vi "Update Plot Name.vi"(8 "error in (no error)":errorcluster, 10 "NewVal":cluster{"String":string, "Picture":picture}[](array[cluster]), 11 "2D Error Bar.lvclass in":refnum<class "2D Error Bar.lvclass">) -> (0 "error out":errorcluster, 3 "2D Error Bar.lvclass out":refnum<class "2D Error Bar.lvclass">)   [LabVIEW 2017, in "2D Error Bar.lvclass"]
uses:
  <vilib>/Math Plots/2D Math Plots/2D Error Bar/2D Error Bar/2D Error Bar.lvclass
  <vilib>/Math Plots/2D Math Plots/2D Error Bar/2D Error Bar/2D Error Bar.lvclass/2D Error Bar.ctl
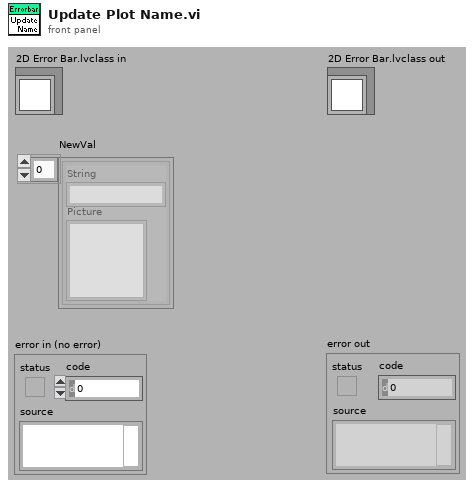
[diagram p1: front panel]
types:
  T1 = typedef "2D Plot.lvclass/Plot Property Array.ctl" = T2[]
  T2 = typedef "2D Plot.lvclass/Plot Property.ctl" = cluster{"Bar Plot Style":u8, "DigitalLineStyle":u8, "TransitionLocation":u8, "Transition Type":u8, "Fill To":i16, "Fill/Pt. Color":u32, "Label Style":u8, "Line Style":u8, "Line Width":u8, "Plot Color":u32, "Plot Interpolation":u8, "Plot Name":string, "Point Style":u8, "Visible?":bool, "XScaleIdx":u32, "YScaleIdx":u32}
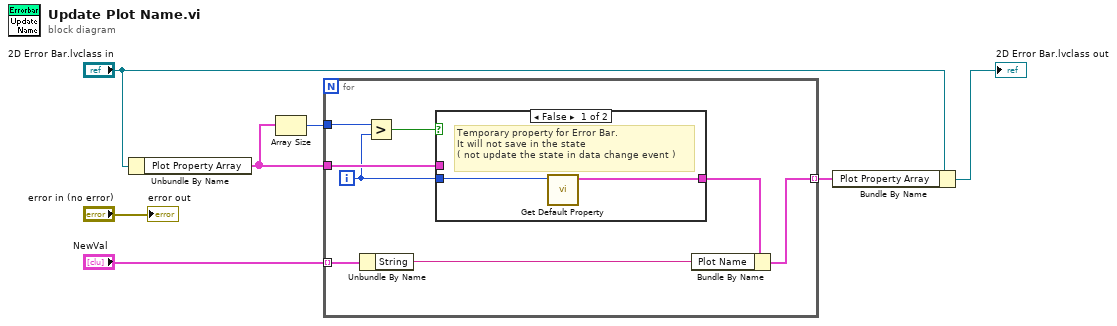
[diagram p0: block diagram]
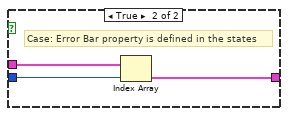
[diagram p2: hidden frame]
diagram:
  n1 = Unbundle By Name("2D Error Bar.lvclass in") -> ("Plot Property Array"=w6:T1)
  n2 = Array Size(array=w6) -> (size(s)=w7:i32)
  n3 = for {
    tunnel: "NewVal" -> [w14] mode=indexing
    tunnel: w6 -> [w10]
    tunnel: [w15] -> w5 mode=indexing
    tunnel: w7 -> [w11]
    i -> [w8]
    n4 = Unbundle By Name(w14) -> ("String"=w13:string)
    n5 = Greater?(x=w11, y=w8) -> (0:w12:bool)
    n6 = case shown="False" w12 {
      tunnel: w10 -> [_ w20]
      tunnel: w8 -> [w17 w19]
      tunnel: [w16 w18] -> w9
      frame False {
        # "Temporary property for Error Bar.\nIt will not save in the state\n( not update the state in data change event )"
        n7 = call <vilib>:"Get Default Property.vi"("Index"=w17) -> ("Temporary Property"=w16:T2)  [unwired: 3 in, 7 out]
      }
      frame True {
        # "Case: Error Bar property is defined in the states"
        n8 = Index Array(array=w20, index=w19) -> (element=w18:T2)
      }
    }
    n9 = Bundle By Name(cluster=w9, "Plot Name"=w13) -> (w15:T2)
  }
  n10 = Bundle By Name(cluster="2D Error Bar.lvclass in", "Plot Property Array"=w5) -> (→"2D Error Bar.lvclass out":refnum<class "2D Error Bar.lvclass">)
  "error out" <- "error in (no error)"
